vi "Main.vi"() -> ()   [LabVIEW 2017]
uses:
  <vilib>/Instr/_visa.llb/VISA Configure Serial Port (Instr).vi
panel:
  in  "VISA resource name":refnum<visa-resource-name>
  out "Longitude [deg]":string
  out "Latitude [deg]":string
  in  "time zone":i32
  out "Time":string
  out "Mode":string
  out "Date [ddmmyy]":string
  out "Course over ground [degrees]":string
  out "Status":string
  out "Speed over ground [knots]":string
  out "E/W":string
  out "Longitude":string
  out "N/S":string
  out "Latitude":string
  out "UTC Time":string
  out "NMEA sentences":string
  in  "[ESC]":bool
  # "GPS demo"
  # "[hhmmss.sss]"
  # "A = vAlid data\nV = inValid data"
  # "[ddmm.mmmm]"
  # "[dddmm.mmmm]"
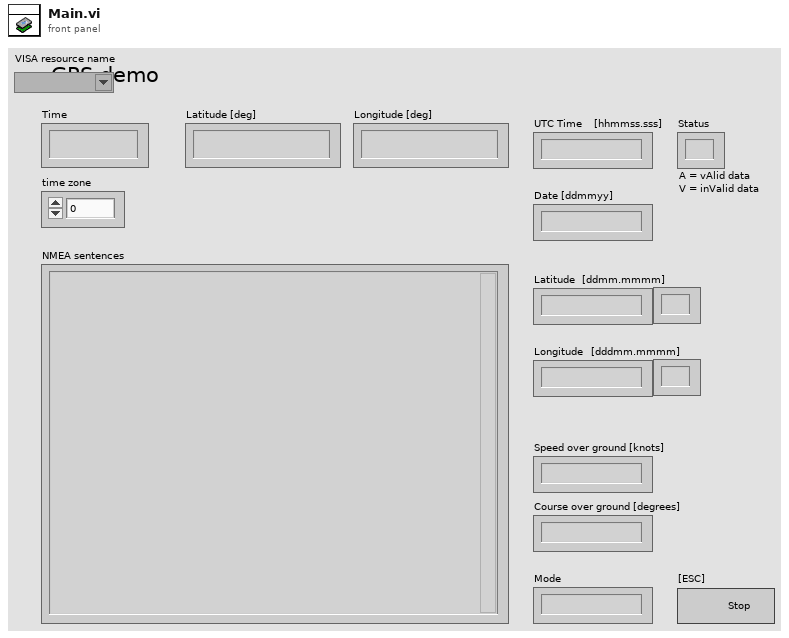
[diagram p1: front panel]
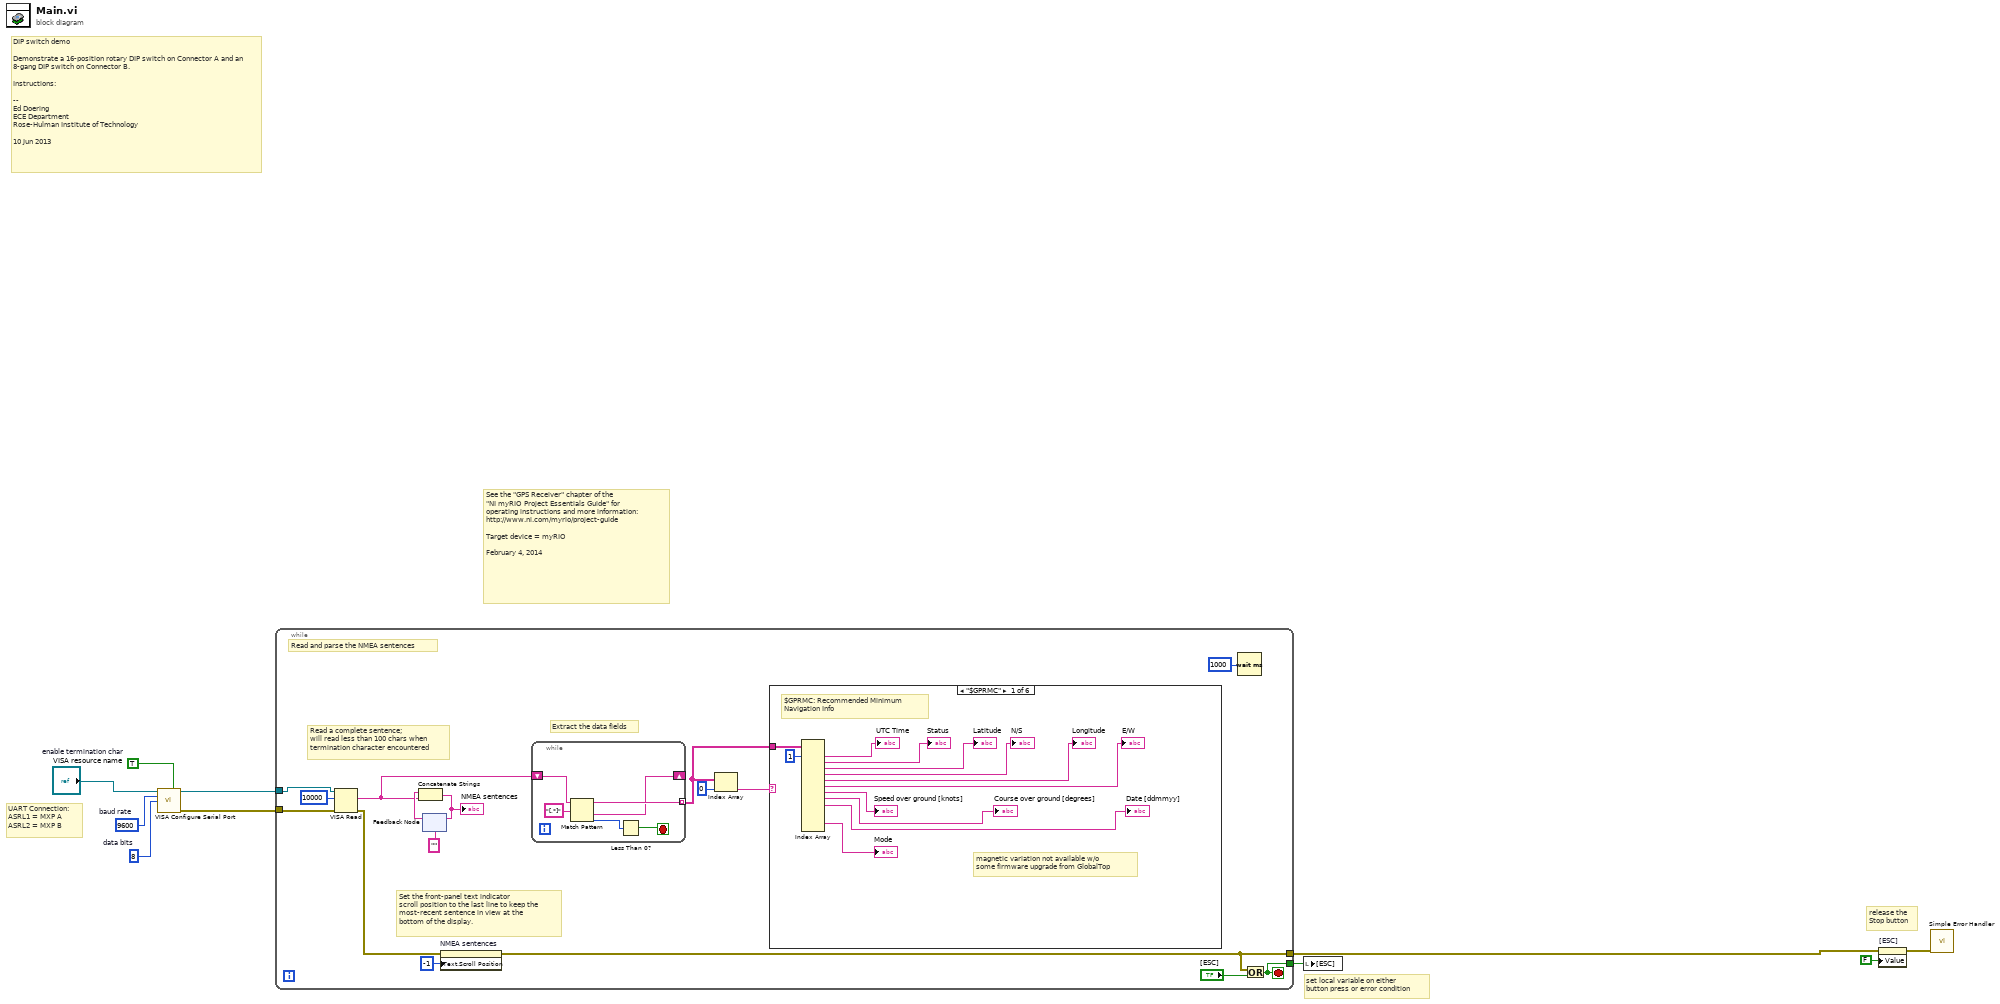
[diagram p0: block diagram]
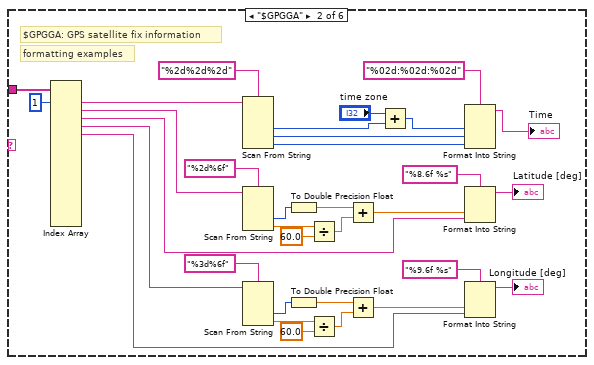
[diagram p2: hidden frame]
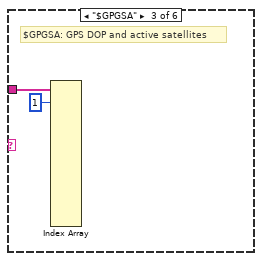
[diagram p3: hidden frame]
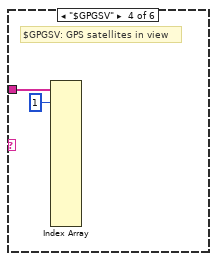
[diagram p4: hidden frame]
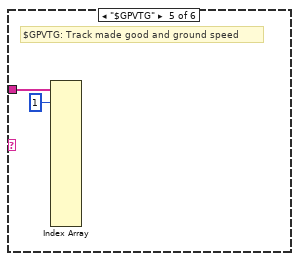
[diagram p5: hidden frame]
diagram:
  w7 = TRUE  # enable termination char
  w8 = u16 8  # data bits
  w9 = u32 9600  # baud rate
  # "See the \"GPS Receiver\" chapter of the\n\"NI myRIO Project Essentials Guide\" for\noperating instructions and more information: \nhttp://www.ni.com/myrio/project-guide\n\nTarget device = myRIO\n\nFebruary 4, 2014"
  # "release the\nStop button"
  # "set local variable on either\nbutton press or error condition"
  # "UART Connection:\nASRL1 = MXP A \nASRL2 = MXP B"
  # "DIP switch demo\n\nDemonstrate a 16-position rotary DIP switch on Connector A and an 8-gang DIP switch on Connector B.\n\nInstructions:\n\n-- \nEd Doering\nECE Department\nRose-Hulman Institute of Technology\n\n10 Jun 2013"
  n1 = call-poly "VISA Configure Serial Port"("VISA resource name"="VISA resource name", "Enable Termination\nChar (T)"=w7, "baud rate (9600)"=w9, "data bits (8)"=w8) -> ("VISA resource name out"=w10:refnum<visa-resource-name>, "error out"=w6:errorcluster)  [unwired: 10 in]
  n2 = while {
    tunnel: [w12] -> w1
    tunnel: w10 -> [w24]
    tunnel: w6 -> [w18]
    tunnel: [w11] -> w5
    stop <- w11 stop-if-true
    # "Set the front-panel text indicator\nscroll position to the last line to keep the\nmost-recent sentence in view at the\nbottom of the display."
    # "Read and parse the NMEA sentences"
    # "Extract the data fields"
    # "Read a complete sentence;\nwill read less than 100 chars when\ntermination character encountered"
    n3 = VISA Read(VISA resource name=w24, byte count=u32 10000, error in (no error)=w18) -> (read buffer=w19:string, error out=w13:errorcluster)  [unwired: 2 out]
    n4 = feedback #1("") -> (w21:string)
    n5 = Concatenate Strings "Concatenate Strings"(w21, w19) -> (w23:string)
    "NMEA sentences" <- w23
    n6 = feedback-in #1(w23) -> ()
    n7 = property on="NMEA sentences" class="Str"(error in=w13, "Text.Scroll Position"=-1) -> (error out=w12:errorcluster)  [unwired: 1 in, 1 out]
    n8 = while {
      tunnel: [w81] -> w16 mode=indexing
      shift-right: [w80] -> _
      shift-left: w19 -> [w82]
      stop <- w79 stop-if-true
      n9 = Match Pattern(string=w82, regular expression="[,*]") -> (before substring=w81:string, after substring=w80:string, offset past match=w78:i32)  [unwired: 1 in, 1 out]
      n10 = Less Than 0?(x=w78) -> (x < 0?=w79:bool)
    }
    n11 = Index Array "Index Array"(array=w16, index=0) -> (element=w17:string)
    n12 = case shown="\"$GPRMC\"" w17 {
      tunnel: w16 -> [w38 w71 w73 w75 w77 _]
      frame "$GPRMC" {
        # "magnetic variation not available w/o\nsome firmware upgrade from GlobalTop"
        # "$GPRMC: Recommended Minimum\nNavigation Info"
        n13 = Index Array "Index Array"(array=w38, index #1=1 ("index")) -> (element #1=→"UTC Time":string, element #2=→"Status":string, element #3=→"Latitude":string, element #4=→"N/S":string, element #5=→"Longitude":string, element #6=→"E/W":string, element #7=→"Speed over ground [knots]":string, element #8=→"Course over ground [degrees]":string, element #9=→"Date [ddmmyy]":string, element #12=→"Mode":string)  [unwired: 12 in, 3 out]
      }
      frame "$GPGGA" {
        # "formatting examples"
        # "$GPGGA: GPS satellite fix information"
        n14 = Index Array "Index Array"(array=w71, index #1=1 ("index")) -> (element #1=w68:string, element #2=w59:string, element #3=w51:string, element #4=w40:string, element #5=w39:string)  [unwired: 15 in, 11 out]
        n15 = Scan From String "Scan From String"(format string="%2d%2d%2d", input string=w68) -> (output 1=w61:i32, output 2=w64:i32, output 3=w66:i32)  [unwired: 5 in, 3 out]
        n16 = Scan From String(format string="%2d%6f", input string=w59) -> (output 1=w56:i32, output 2=w58:dbl)  [unwired: 4 in, 3 out]
        n17 = Scan From String(format string="%3d%6f", input string=w40) -> (output 1=w44:i32, output 2=w42:dbl)  [unwired: 4 in, 3 out]
        n18 = To Double Precision Float(number=w56) -> (double precision float=w54:dbl)
        n19 = To Double Precision Float(number=w44) -> (double precision float=w46:dbl)
        n20 = Divide(x=w58, y=60.0) -> (x/y=w55:dbl)
        n21 = Divide(x=w42, y=60.0) -> (x/y=w45:dbl)
        n22 = Add(x=w54, y=w55) -> (x+y=w52:dbl)
        n23 = Add(x=w46, y=w45) -> (x+y=w48:dbl)
        n24 = Add(x="time zone", y=w61) -> (x+y=w62:i32)
        n25 = Format Into String "Format Into String"(format string="%02d:%02d:%02d", w62, w64, w66) -> (resulting string=→"Time":string)  [unwired: 2 in, 1 out]
        n26 = Format Into String(format string="%8.6f %s", w52, w51) -> (resulting string=→"Latitude [deg]":string)  [unwired: 2 in, 1 out]
        n27 = Format Into String(format string="%9.6f %s", w48, w39) -> (resulting string=→"Longitude [deg]":string)  [unwired: 2 in, 1 out]
      }
      frame "$GPGSA" {
        # "$GPGSA: GPS DOP and active satellites"
        n28 = Index Array(array=w73, index #1=1 ("index")) -> ()  [unwired: 15 in, 16 out]
      }
      frame "$GPGSV" {
        # "$GPGSV: GPS satellites in view"
        n29 = Index Array(array=w75, index #1=1 ("index")) -> ()  [unwired: 15 in, 16 out]
      }
      frame "$GPVTG" {
        # "$GPVTG: Track made good and ground speed"
        n30 = Index Array(array=w77, index #1=1 ("index")) -> ()  [unwired: 15 in, 16 out]
      }
      frame Default {
      }
    }
    n31 = Wait (ms)(milliseconds to wait=u32 1000) -> ()  [unwired: 1 out]
    n32 = Or(x=w12, y="[ESC]") -> (x .or. y?=w11:bool)
  }
  n33 = local write "[ESC]"(w5) -> ()
  n34 = property on="[ESC]" class="Bool (strict)"(error in=w1, "Value"=FALSE ("[ESC]")) -> (error out=w3:errorcluster)  [unwired: 1 in, 1 out]
  n35 = call <vilib>:"Simple Error Handler.vi"("error in (no error)"=w3) -> ()  [unwired: 4 in, 5 out]
